vi "2d_array.vi"() -> ()   [LabVIEW 2017]
uses:
  measurement_data/MeasurementDatalvclass.lvclass
  support/my_global.vi
panel:
  out "output":u16[](array[numeric])
  out "size(s)":i32[](array[numeric])
  out "Array":dbl[][](array[numeric])
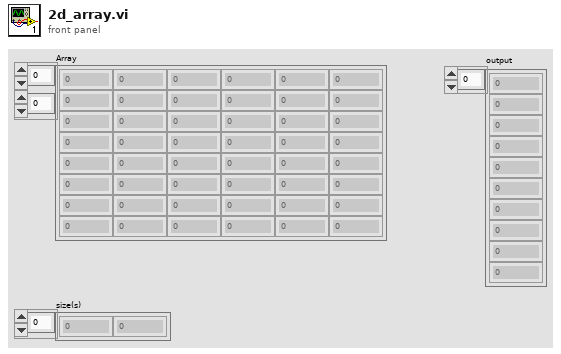
[diagram p1: front panel]
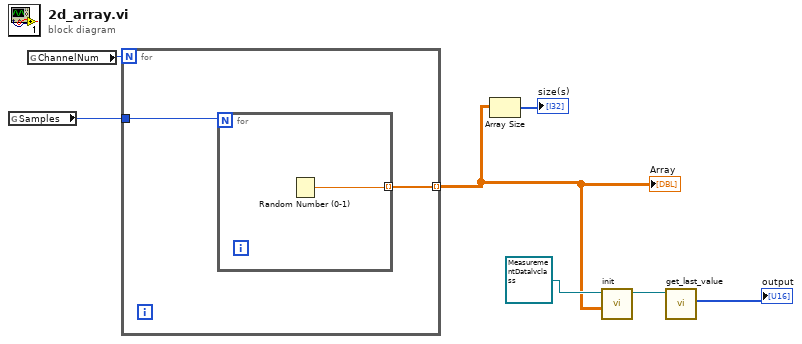
[diagram p0: block diagram]
diagram:
  n1 = global read "my_global.vi" "Samples"() -> (w5:u32)
  n2 = global read "my_global.vi" "ChannelNum"() -> (w6:u32)
  n3 = for {
    N: w6 -> [_]
    tunnel: [w9] -> w3 mode=indexing
    tunnel: w5 -> [w8]
    n4 = for {
      N: w8 -> [_]
      tunnel: [w10] -> w9 mode=indexing
      n5 = Random Number (0-1)() -> (number: 0 to 1=w10:dbl)
    }
  }
  "Array" <- w3
  n6 = Array Size(array=w3) -> (size(s)=→"size(s)":i32[])
  n7 = call-dynamic "init.vi"("inputs"=w3, "MeasurementResult in"=refnum<class "MeasurementDatalvclass.lvclass"> refnum ("MeasurementDatalvclass.lvclass")) -> ("MeasurementResult out"=w2:refnum<class "MeasurementDatalvclass.lvclass">)  [unwired: 8 in, 1 out]
  n8 = call "get_last_value.vi"("MeasurementDatalvclass in"=w2) -> ("output"=→"output":u16[])  [unwired: 8 in, 2 out]
